vi "ScanSteuerung_to_Datapoints_Transposed.vi"(2 "Datapoints (-1=estimate)":i32=-1, 3 "ScanSteuerung":T3(array[cluster])=[{"Zeitpunkt [s]"=0.0, "Wirkung"=enum."Abs", "Kanal"=enum."GalvoX", "Wert (/s)"=-8.3466666667e-05}, {"Zeitpunkt [s]"=0.0, "Wirkung"=enum."Abs", "Kanal"=enum."GalvoY", "Wert (/s)"=6.7466666667e-05}, {"Zeitpunkt [s]"=0.0, "Wirkung"=enum."Inc", "Kanal"=enum."GalvoX", "Wert (/s)"=0.0888}, {"Zeitpunkt [s]"=0.0, "Wirkung"=enum."Inc", "Kanal"=enum."GalvoY", "Wert (/s)"=0.0}, {"Zeitpunkt [s]"=0.00119, "Wirkung"=enum."LoopStart", "Kanal"=enum."Loop", "Wert (/s)"=4.0}, {"Zeitpunkt [s]"=0.00119, "Wirkung"=enum."Abs", "Kanal"=enum."Digital", "Wert (/s)"=7.0}, {"Zeitpunkt [s]"=0.002, "Wirkung"=enum."Inc", "Kanal"=enum."GalvoX", "Wert (/s)"=-3.3095271315e-17}, {"Zeitpunkt [s]"=0.002, "Wirkung"=enum."Inc", "Kanal"=enum."GalvoY", "Wert (/s)"=-0.0818}, {"Zeitpunkt [s]"=0.0022, "Wirkung"=enum."Inc", "Kanal"=enum."GalvoX", "Wert (/s)"=-0.0888}, {"Zeitpunkt [s]"=0.0022, "Wirkung"=enum."Inc", "Kanal"=enum."GalvoY", "Wert (/s)"=0.0}, {"Zeitpunkt [s]"=0.00319, "Wirkung"=enum."Abs", "Kanal"=enum."Digital", "Wert (/s)"=5.0}, {"Zeitpunkt [s]"=0.0033900000000000002, "Wirkung"=enum."Abs", "Kanal"=enum."Digital", "Wert (/s)"=7.0}, {"Zeitpunkt [s]"=0.0042, "Wirkung"=enum."Inc", "Kanal"=enum."GalvoX", "Wert (/s)"=3.3095271315e-17}, {"Zeitpunkt [s]"=0.0042, "Wirkung"=enum."Inc", "Kanal"=enum."GalvoY", "Wert (/s)"=-0.0818}, {"Zeitpunkt [s]"=0.0044, "Wirkung"=enum."Inc", "Kanal"=enum."GalvoX", "Wert (/s)"=0.0888}, {"Zeitpunkt [s]"=0.0044, "Wirkung"=enum."Inc", "Kanal"=enum."GalvoY", "Wert (/s)"=0.0}, {"Zeitpunkt [s]"=0.00539, "Wirkung"=enum."Abs", "Kanal"=enum."Digital", "Wert (/s)"=5.0}, {"Zeitpunkt [s]"=0.00559, "Wirkung"=enum."LoopEnd", "Kanal"=enum."Loop", "Wert (/s)"=0.0}, {"Zeitpunkt [s]"=0.01879, "Wirkung"=enum."Abs", "Kanal"=enum."Digital", "Wert (/s)"=7.0}, {"Zeitpunkt [s]"=0.0196, "Wirkung"=enum."Inc", "Kanal"=enum."GalvoX", "Wert (/s)"=-3.3095271315e-17}, {"Zeitpunkt [s]"=0.0196, "Wirkung"=enum."Inc", "Kanal"=enum."GalvoY", "Wert (/s)"=-0.0818}, {"Zeitpunkt [s]"=0.0198, "Wirkung"=enum."Inc", "Kanal"=enum."GalvoX", "Wert (/s)"=-0.0888}, {"Zeitpunkt [s]"=0.0198, "Wirkung"=enum."Inc", "Kanal"=enum."GalvoY", "Wert (/s)"=0.0}, {"Zeitpunkt [s]"=0.02079, "Wirkung"=enum."Abs", "Kanal"=enum."Digital", "Wert (/s)"=5.0}, {"Zeitpunkt [s]"=0.02099, "Wirkung"=enum."Abs", "Kanal"=enum."Digital", "Wert (/s)"=7.0}, {"Zeitpunkt [s]"=0.0218, "Wirkung"=enum."Inc", "Kanal"=enum."GalvoX", "Wert (/s)"=0.0}, {"Zeitpunkt [s]"=0.0218, "Wirkung"=enum."Inc", "Kanal"=enum."GalvoY", "Wert (/s)"=0.0}, {"Zeitpunkt [s]"=0.0218, "Wirkung"=enum."LoopStart", "Kanal"=enum."Loop", "Wert (/s)"=2.0}, {"Zeitpunkt [s]"=0.021810000000000003, "Wirkung"=enum."Abs", "Kanal"=enum."GalvoX", "Wert (/s)"=-8.3466666667e-05}, {"Zeitpunkt [s]"=0.021810000000000003, "Wirkung"=enum."Abs", "Kanal"=enum."GalvoY", "Wert (/s)"=6.7466666667e-05}, {"Zeitpunkt [s]"=0.021810000000000003, "Wirkung"=enum."Inc", "Kanal"=enum."GalvoX", "Wert (/s)"=0.0888}, {"Zeitpunkt [s]"=0.021810000000000003, "Wirkung"=enum."Inc", "Kanal"=enum."GalvoY", "Wert (/s)"=0.0}, {"Zeitpunkt [s]"=0.023000000000000003, "Wirkung"=enum."LoopStart", "Kanal"=enum."Loop", "Wert (/s)"=4.0}, {"Zeitpunkt [s]"=0.023000000000000003, "Wirkung"=enum."Abs", "Kanal"=enum."Digital", "Wert (/s)"=7.0}, {"Zeitpunkt [s]"=0.023810000000000005, "Wirkung"=enum."Inc", "Kanal"=enum."GalvoX", "Wert (/s)"=-3.3095271315e-17}, {"Zeitpunkt [s]"=0.023810000000000005, "Wirkung"=enum."Inc", "Kanal"=enum."GalvoY", "Wert (/s)"=-0.0818}, {"Zeitpunkt [s]"=0.024010000000000004, "Wirkung"=enum."Inc", "Kanal"=enum."GalvoX", "Wert (/s)"=-0.0888}, {"Zeitpunkt [s]"=0.024010000000000004, "Wirkung"=enum."Inc", "Kanal"=enum."GalvoY", "Wert (/s)"=0.0}, {"Zeitpunkt [s]"=0.025, "Wirkung"=enum."Abs", "Kanal"=enum."Digital", "Wert (/s)"=5.0}, {"Zeitpunkt [s]"=0.025200000000000004, "Wirkung"=enum."Abs", "Kanal"=enum."Digital", "Wert (/s)"=7.0}, {"Zeitpunkt [s]"=0.026010000000000002, "Wirkung"=enum."Inc", "Kanal"=enum."GalvoX", "Wert (/s)"=3.3095271315e-17}, {"Zeitpunkt [s]"=0.026010000000000002, "Wirkung"=enum."Inc", "Kanal"=enum."GalvoY", "Wert (/s)"=-0.0818}, {"Zeitpunkt [s]"=0.026210000000000004, "Wirkung"=enum."Inc", "Kanal"=enum."GalvoX", "Wert (/s)"=0.0888}, {"Zeitpunkt [s]"=0.026210000000000004, "Wirkung"=enum."Inc", "Kanal"=enum."GalvoY", "Wert (/s)"=0.0}, {"Zeitpunkt [s]"=0.027200000000000002, "Wirkung"=enum."Abs", "Kanal"=enum."Digital", "Wert (/s)"=5.0}, {"Zeitpunkt [s]"=0.027400000000000004, "Wirkung"=enum."LoopEnd", "Kanal"=enum."Loop", "Wert (/s)"=0.0}, {"Zeitpunkt [s]"=0.040600000000000004, "Wirkung"=enum."Abs", "Kanal"=enum."Digital", "Wert (/s)"=7.0}, {"Zeitpunkt [s]"=0.04141, "Wirkung"=enum."Inc", "Kanal"=enum."GalvoX", "Wert (/s)"=-3.3095271315e-17}, {"Zeitpunkt [s]"=0.04141, "Wirkung"=enum."Inc", "Kanal"=enum."GalvoY", "Wert (/s)"=-0.0818}, {"Zeitpunkt [s]"=0.04161000000000001, "Wirkung"=enum."Inc", "Kanal"=enum."GalvoX", "Wert (/s)"=-0.0888}, {"Zeitpunkt [s]"=0.04161000000000001, "Wirkung"=enum."Inc", "Kanal"=enum."GalvoY", "Wert (/s)"=0.0}, {"Zeitpunkt [s]"=0.0426, "Wirkung"=enum."Abs", "Kanal"=enum."Digital", "Wert (/s)"=5.0}, {"Zeitpunkt [s]"=0.042800000000000005, "Wirkung"=enum."Abs", "Kanal"=enum."Digital", "Wert (/s)"=7.0}, {"Zeitpunkt [s]"=0.04361, "Wirkung"=enum."Inc", "Kanal"=enum."GalvoX", "Wert (/s)"=0.0}, {"Zeitpunkt [s]"=0.04361, "Wirkung"=enum."Inc", "Kanal"=enum."GalvoY", "Wert (/s)"=0.0}, {"Zeitpunkt [s]"=0.044789999999999996, "Wirkung"=enum."Abs", "Kanal"=enum."Digital", "Wert (/s)"=4.0}, {"Zeitpunkt [s]"=0.044800000000000006, "Wirkung"=enum."Abs", "Kanal"=enum."Digital", "Wert (/s)"=4.0}, {"Zeitpunkt [s]"=0.04361, "Wirkung"=enum."LoopEnd", "Kanal"=enum."Loop", "Wert (/s)"=0.0}, {"Zeitpunkt [s]"=0.06661, "Wirkung"=enum."Abs", "Kanal"=enum."Digital", "Wert (/s)"=0.0}], 4 "Aktiv":T2(array[ring])=[enum."GalvoX", enum."GalvoY"], 5 "Neues Zeitraster":dbl=1e-05) -> (0 "ScanSteuerungOut":T1(array[cluster])=[{"Zeitpunkt [s]"=0.0, "Wirkung"=enum."Abs", "Kanal"=0.0, "Wert (/s)"=0.0}, {"Zeitpunkt [s]"=0.0, "Wirkung"=enum."Inc", "Kanal"=0.0, "Wert (/s)"=0.0001}, {"Zeitpunkt [s]"=0.0, "Wirkung"=enum."Abs", "Kanal"=1.0, "Wert (/s)"=0.5}, {"Zeitpunkt [s]"=0.0, "Wirkung"=enum."IncInc", "Kanal"=0.0, "Wert (/s)"=-1.0000000000000002e-08}, {"Zeitpunkt [s]"=0.0, "Wirkung"=enum."IncInc", "Kanal"=1.0, "Wert (/s)"=-1.0000000000000002e-08}, {"Zeitpunkt [s]"=10000.0, "Wirkung"=enum."IncInc", "Kanal"=1.0, "Wert (/s)"=1.0000000000000002e-08}, {"Zeitpunkt [s]"=20000.0, "Wirkung"=enum."IncInc", "Kanal"=0.0, "Wert (/s)"=1.0000000000000002e-08}, {"Zeitpunkt [s]"=29999.999999999996, "Wirkung"=enum."IncInc", "Kanal"=1.0, "Wert (/s)"=-1.0000000000000002e-08}, {"Zeitpunkt [s]"=40000.0, "Wirkung"=enum."IncInc", "Kanal"=0.0, "Wert (/s)"=0.0}], 1 "Waveform Graph":dbl[][](graph))   [LabVIEW 2011]
panel:
  out "wrong command oder - STOP":bool
  out "Datapoints":i32=40001
  # "Transposed Datapoints!"
  # "After the loop there has to be at lest one datapoint in one activ channel\nOrder: add abs and rel-values, generate pint, add inc, add incinc to inc\ne.g. at t there is inc: t+1 there is the second pont (t,t+1) with one inc!"
  # "now with incinc support!\nnow with nested loops support!"
  # "Error handling for wrong loops!\nbut there is no error out"
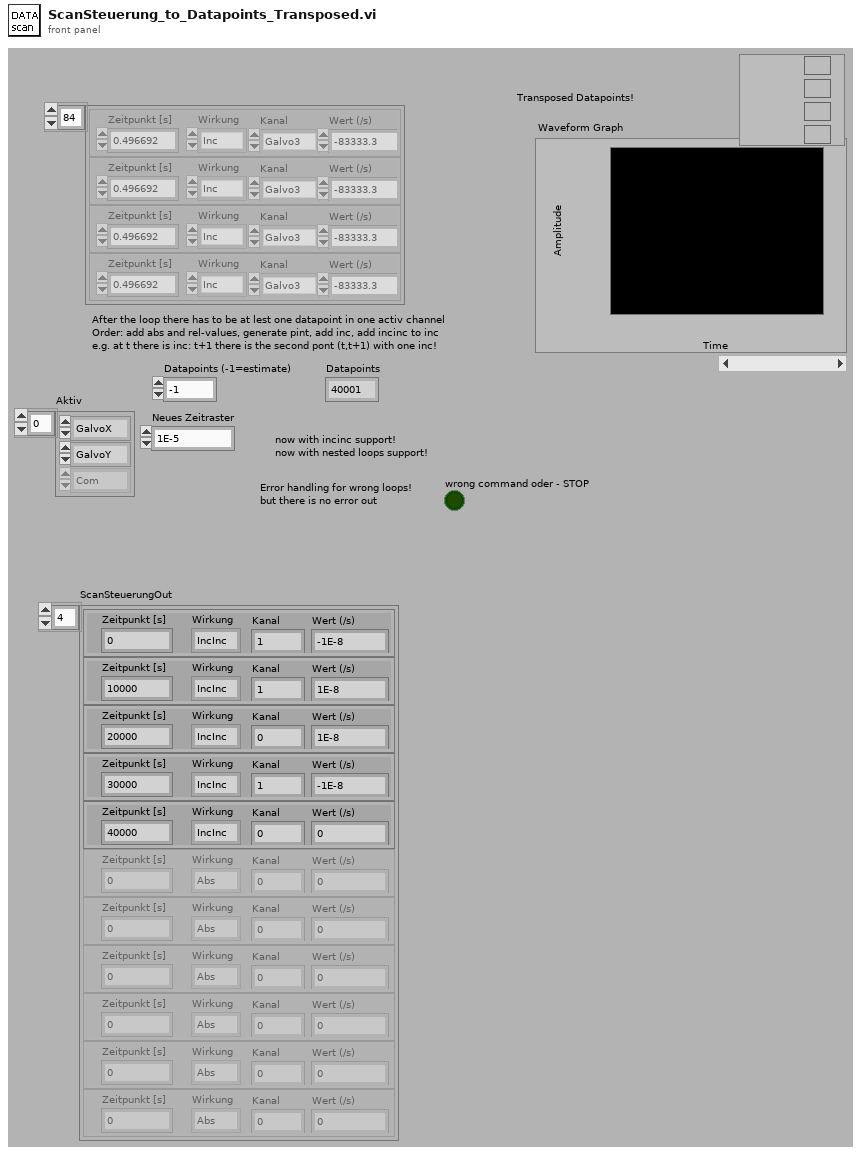
[diagram p1: front panel]
types:
  T1 = cluster{"Zeitpunkt [s]":dbl, "Wirkung":enum16{"Abs", "Rel", "Inc", "IncInc", "LoopStart", "LoopEnd"}, "Kanal":dbl, "Wert (/s)":dbl}[]
  T2 = enum16{"Com", "AnalogConfig", "AnalogValue", "GalvoX", "GalvoY", "Galvo3", "Galvo4", "Digital", "Free", "Loop", "SMoveTime", "Image1X", "Image1Y", "Image2X", "Image2Y"}[]
  T3 = cluster{"Zeitpunkt [s]":dbl, "Wirkung":enum16{"Abs", "Rel", "Inc", "IncInc", "LoopStart", "LoopEnd"}, "Kanal":enum16{"Com", "AnalogConfig", "AnalogValue", "GalvoX", "GalvoY", "Galvo3", "Galvo4", "Digital", "Free", "Loop", "SMoveTime", "Image1X", "Image1Y", "Image2X", "Image2Y"}, "Wert (/s)":dbl}[]
  T4 = cluster{"Time offsets":i32[], "Array":cluster{"Loopstart#":u32, "Loops to do":i32}[]}
  T5 = typedef "ScanControl.ctl" = cluster{"Time [s]":dbl, "action":T6, "channel":T7, "value (/s)":dbl}[]
  T6 = typedef "ScanControl_Action.ctl" = enum16{"Abs", "Rel", "Inc", "IncInc", "LoopStart", "LoopEnd", "WaitTriggerRising"}
  T7 = typedef "ScanControl_Channel.ctl" = enum16{"Com", "AnalogConfig", "AnalogValue", "GalvoX", "GalvoY", "Galvo3", "Galvo4", "Digital", "Free", "Loop", "SMoveTime", "Image1X", "Image1Y", "Image2X", "Image2Y"}
  T8 = cluster{"Zeitpunkt [s]":dbl, "Wirkung":enum16{"Abs", "Rel", "Inc", "IncInc", "LoopStart", "LoopEnd"}, "Kanal":i32, "Wert (/s)":dbl}[]
  T9 = cluster{"Zeitpunkt [s]":dbl, "Wirkung":enum16{"Abs", "Rel", "Inc", "IncInc", "LoopStart", "LoopEnd"}, "Kanal":i32, "Wert (/s)":dbl}
  T10 = enum16{"Abs", "Rel", "Inc", "IncInc", "LoopStart", "LoopEnd"}
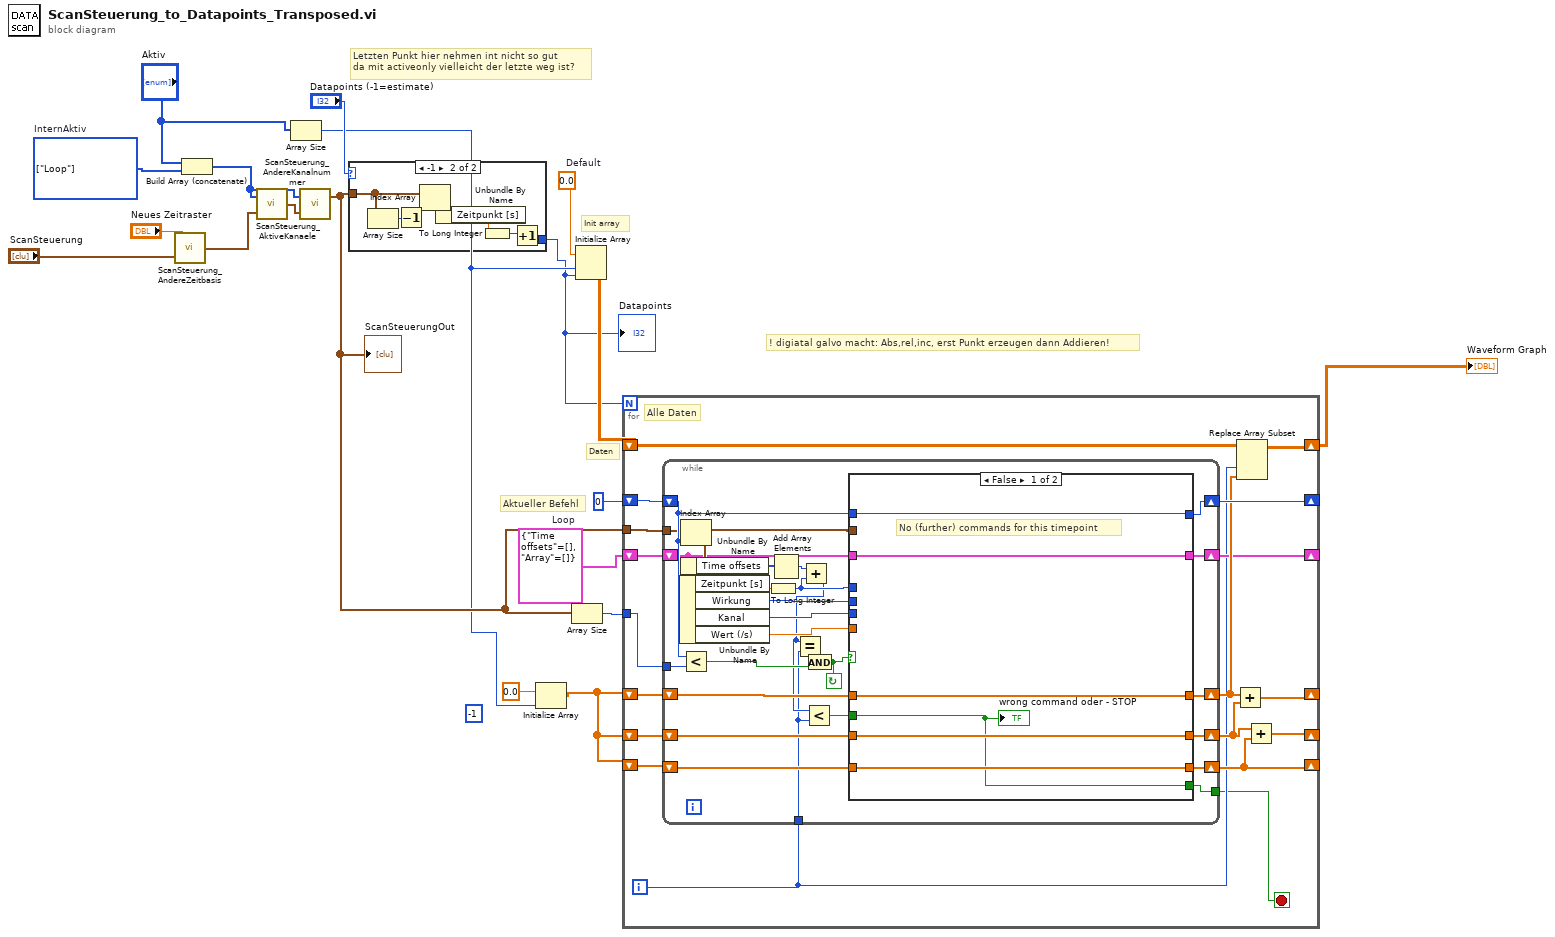
[diagram p0: block diagram]
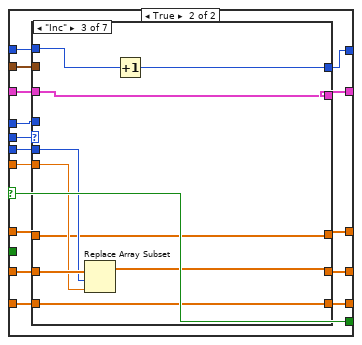
[diagram p3: hidden frame]
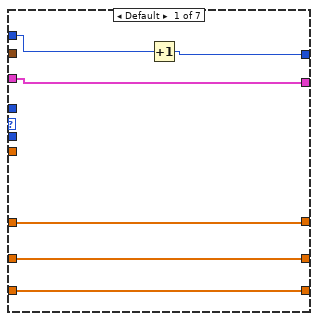
[diagram p4: hidden frame]
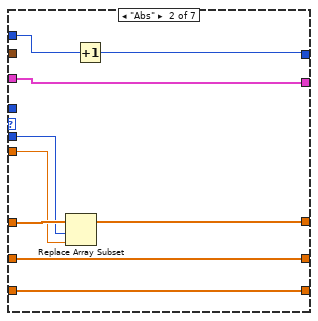
[diagram p5: hidden frame]
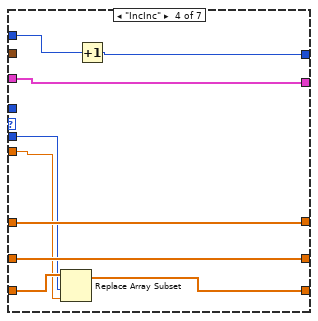
[diagram p6: hidden frame]
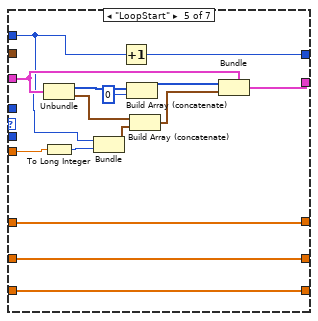
[diagram p7: hidden frame]
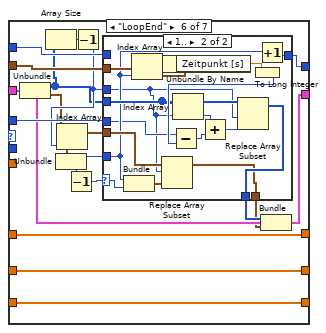
[diagram p8: hidden frame]
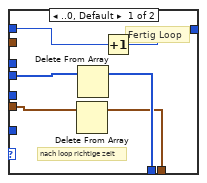
[diagram p9: hidden frame]
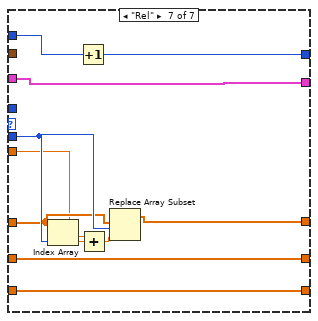
[diagram p10: hidden frame]
diagram:
  (unwired) -1 ("LoopLevel")
  w3 = T4 {"Time offsets"=[], "Array"=[]}  # Loop
  w12 = T2 [enum."Loop"] items=["Com", "AnalogConfig", "AnalogValue", "GalvoX", "GalvoY", "Galvo3", "Galvo4", "Digital", "Free", "Loop", "SMoveTime", "Image1X", "Image1Y", "Image2X", "Image2Y"]  # InternAktiv
  w19 = 0.0  # Default
  # "! digiatal galvo macht: Abs,rel,inc, erst Punkt erzeugen dann Addieren!"
  # "Letzten Punkt hier nehmen int nicht so gut\nda mit activeonly vielleicht der letzte weg ist?"
  # "Aktueller Befehl"
  # "Daten"
  # "Init array"
  n1 = call "ScanSteuerung_AndereZeitbasis.vi"("ScanSteuerung"="ScanSteuerung", "Neues Zeitraster"="Neues Zeitraster") -> ("ScanSteuerungOut"=w9:T5)
  n2 = Build Array (concatenate)("Aktiv", w12) -> (w10:T2)
  n3 = call "ScanSteuerung_AktiveKanaele.vi"("ScanSteuerung"=w9, "Aktiv"=w10) -> ("ScanSteuerungOut"=w14:T5)
  n4 = Array Size(array="Aktiv") -> (size(s)=w2:i32)
  n5 = call "ScanSteuerung_AndereKanalnummer.vi"("ScanSteuerung"=w14, "Neue Kanalnummer (nicht gefunden gibt 0!)"=w10) -> ("ScanSteuerungOut"=w13:T8)  [unwired: 1 out]
  "ScanSteuerungOut" <- w13
  n6 = case shown="-1" "Datapoints (-1=estimate)" {
    selector: "Datapoints (-1=estimate)" -> [w20 _]
    tunnel: w13 -> [_ w23]
    tunnel: [w20 w21] -> w1
    frame 0, Default {
    }
    frame -1 {
      n7 = Array Size(array=w23) -> (size(s)=w27:i32)
      n8 = Decrement(x=w27) -> (x-1=w26:i32)
      n9 = Index Array(array=w23, index=w26) -> (element=w25:T9)
      n10 = Unbundle By Name(w25) -> ("Zeitpunkt [s]"=w24:dbl)
      n11 = To Long Integer(number=w24) -> (32bit integer=w22:i32)
      n12 = Increment(x=w22) -> (x+1=w21:i32)
    }
  }
  "Datapoints" <- w1
  n13 = Initialize Array(0.0 ("element"), w2) -> (w4:dbl[])
  n14 = Array Size(array=w13) -> (size(s)=w16:i32)
  n15 = Initialize Array(w19, w2, w1) -> (w17:dbl[][])
  n16 = for {
    N: w1 -> [_]
    shift-left: w4 -> [w43]
    shift-right: [w39] -> _
    tunnel: w16 -> [w37]
    shift-left: u32 0 -> [w44]
    shift-right: [w38] -> _
    shift-left: w17 -> [w41]
    shift-right: [w40] -> w7
    tunnel: w13 -> [w45]
    shift-right: [w34] -> _
    shift-left: w4 -> [w42]
    shift-right: [w32] -> _
    shift-left: w4 -> [w35]
    shift-right: [w30] -> _
    shift-left: w3 -> [w31]
    i -> [w29]
    stop <- w28 stop-if-true
    # "Alle Daten"
    n17 = while {
      tunnel: w45 -> [w54]
      shift-right: [w64] -> w38
      shift-left: w44 -> [w61]
      shift-right: [w67] -> w36
      shift-left: w43 -> [w71]
      shift-right: [w66] -> w33
      shift-left: w42 -> [w70]
      tunnel: w29 -> [w48]
      tunnel: w37 -> [w60]
      shift-right: [w55] -> w32
      shift-left: w35 -> [w56]
      shift-right: [w52] -> w30
      shift-left: w31 -> [w53]
      tunnel: [w46] -> w28
      stop <- w57 continue-if-true
      n18 = Index Array(array=w54, index=w61) -> (element=w72:T9)
      n19 = Unbundle By Name(w72) -> ("Zeitpunkt [s]"=w63:dbl, "Wirkung"=w65:T10, "Kanal"=w69:i32, "Wert (/s)"=w68:dbl)
      n20 = Unbundle By Name(w53) -> ("Time offsets"=w51:i32[])
      n21 = Less?(x=w61, y=w60) -> (x < y?=w58:bool)
      n22 = To Long Integer(number=w63) -> (32bit integer=w62:i32)
      n23 = Add Array Elements(numeric array=w51) -> (sum=w50:i32)
      n24 = Add(x=w50, y=w62) -> (x+y=w49:i32)
      n25 = Equal?(x=w49, y=w48) -> (x = y?=w59:bool)
      n26 = Less?(x=w49, y=w48) -> (x < y?=w47:bool)
      n27 = And(x=w59, y=w58) -> (x .and. y?=w57:bool)
      n28 = case shown="False" w57 {
        selector: w57 -> [_ w79]
        tunnel: w71 -> [w78 w94]
        tunnel: w70 -> [w77 w93]
        tunnel: w69 -> [_ w92]
        tunnel: w68 -> [_ w91]
        tunnel: [w78 w90] -> w67
        tunnel: [w77 w89] -> w66
        tunnel: w65 -> [_ w88]
        tunnel: w61 -> [w76 w87]
        tunnel: [w76 w86] -> w64
        tunnel: w62 -> [_ w85]
        tunnel: w56 -> [w75 w84]
        tunnel: [w75 w83] -> w55
        tunnel: w54 -> [_ w82]
        tunnel: w53 -> [w74 w81]
        tunnel: [w74 w80] -> w52
        tunnel: w47 -> [w73 _]
        tunnel: [w73 w79] -> w46
        frame False {
          # "No (further) commands for this timepoint"
          "wrong command oder - STOP" <- w73
        }
        frame True {
          n29 = case shown="\"Inc\"" w88 {
            tunnel: w94 -> [w98 w109 w114 w127 w142 w161 w192]
            tunnel: w93 -> [w97 w105 w118 w126 w141 w160 w191]
            tunnel: w92 -> [_ w108 w116 w122 _ _ w193]
            tunnel: w91 -> [_ w107 w115 w121 w140 _ w190]
            tunnel: [w98 w106 w114 w127 w142 w161 w195] -> w90
            tunnel: [w97 w105 w117 w126 w141 w160 w191] -> w89
            tunnel: w87 -> [w100 w104 w113 w125 w135 w158 w188]
            tunnel: [w95 w103 w112 w124 w139 w159 w187] -> w86
            tunnel: w85 -> [_ _ _ _ _ w157 _]
            tunnel: w84 -> [w96 w102 w111 w123 w138 w156 w186]
            tunnel: [w96 w102 w111 w120 w138 w156 w186] -> w83
            tunnel: w82 -> [_ _ _ _ _ w155 _]
            tunnel: w81 -> [w99 w101 w110 w119 w136 w151 w185]
            tunnel: [w99 w101 w110 w119 w137 w152 w185] -> w80
            frame Default {
              n30 = Increment(x=w100) -> (x+1=w95:u32)
            }
            frame "Abs" {
              n31 = Replace Array Subset(array=w109, new element=w107, index=w108) -> (w106:dbl[])
              n32 = Increment(x=w104) -> (x+1=w103:u32)
            }
            frame "Inc" {
              n33 = Replace Array Subset(array=w118, new element=w115, index=w116) -> (w117:dbl[])
              n34 = Increment(x=w113) -> (x+1=w112:u32)
            }
            frame "IncInc" {
              n35 = Replace Array Subset(array=w123, new element=w121, index=w122) -> (w120:dbl[])
              n36 = Increment(x=w125) -> (x+1=w124:u32)
            }
            frame "LoopStart" {
              n37 = Unbundle(w136) -> ("Time offsets"=w129:i32[], "Array"=w128:cluster{"Loopstart#":u32, "Loops to do":i32}[])
              n38 = To Long Integer(number=w140) -> (32bit integer=w134:i32)
              n39 = Bundle(w135, w134) -> (w132:cluster{u32, i32})  [unwired: 1 out]
              n40 = Increment(x=w135) -> (x+1=w139:u32)
              n41 = Build Array (concatenate)(w129, 0) -> (w131:i32[])
              n42 = Build Array (concatenate)(w128, w132) -> (w133:cluster{"Loopstart#":u32, "Loops to do":i32}[])
              n43 = Bundle(cluster=w136, "Time offsets"=w131, "Array"=w133) -> (w137:T4)
            }
            frame "LoopEnd" {
              n44 = Unbundle(w151) -> ("Time offsets"=w144:i32[], "Array"=w143:cluster{"Loopstart#":u32, "Loops to do":i32}[])
              n45 = Array Size(array=w144) -> (size(s)=w146:i32)
              n46 = Decrement(x=w146) -> (x-1=w145:i32)
              n47 = Index Array(array=w143, index=w145) -> (element=w150:cluster{"Loopstart#":u32, "Loops to do":i32})
              n48 = Unbundle(w150) -> ("Loopstart#"=w153:u32, "Loops to do"=w154:i32)
              n49 = Decrement(x=w154) -> (x-1=w149:i32)
              n50 = case shown="1.." w149 {
                selector: w149 -> [_ w171]
                tunnel: w144 -> [w165 w175]
                tunnel: [w166 w184] -> w159
                tunnel: w158 -> [w167 _]
                tunnel: w157 -> [_ w169]
                tunnel: w155 -> [_ w182]
                tunnel: w153 -> [_ w170]
                tunnel: w145 -> [_ w168]
                tunnel: [w164 w176] -> w148
                tunnel: w143 -> [w163 w173]
                tunnel: [w162 w174] -> w147
                frame ..0, Default {
                  # "nach loop richtige zeit"
                  # "Fertig Loop"
                  n51 = Delete From Array(array=w163) -> (array with subset deleted=w162:cluster{"Loopstart#":u32, "Loops to do":i32}[])  [unwired: 2 in, 1 out]
                  n52 = Delete From Array(array=w165) -> (array with subset deleted=w164:i32[])  [unwired: 2 in, 1 out]
                  n53 = Increment(x=w167) -> (x+1=w166:u32)
                }
                frame 1.. {
                  n54 = Bundle("Loopstart#"=w170, w171) -> (w172:cluster{"Loopstart#":u32, i32})  [unwired: 1 out]
                  n55 = Index Array(array=w182, index=w170) -> (element=w181:T9)
                  n56 = Unbundle By Name(w181) -> ("Zeitpunkt [s]"=w180:dbl)
                  n57 = Replace Array Subset(array=w173, new element=w172, index=w168) -> (w174:cluster{"Loopstart#":u32, "Loops to do":i32}[])
                  n58 = Index Array(array=w175, index=w168) -> (element=w178:i32)
                  n59 = To Long Integer(number=w180) -> (32bit integer=w179:i32)
                  n60 = Subtract(x=w169, y=w179) -> (x-y=w183:i32)
                  n61 = Add(x=w178, y=w183) -> (x+y=w177:i32)
                  n62 = Replace Array Subset(array=w175, new element=w177, index=w168) -> (w176:i32[])
                  n63 = Increment(x=w170) -> (x+1=w184:u32)
                }
              }
              n64 = Bundle(cluster=w151, "Time offsets"=w148, "Array"=w147) -> (w152:T4)
            }
            frame "Rel" {
              n65 = Index Array(array=w192, index=w193) -> (element=w189:dbl)
              n66 = Increment(x=w188) -> (x+1=w187:u32)
              n67 = Add(x=w190, y=w189) -> (x+y=w194:dbl)
              n68 = Replace Array Subset(array=w192, new element=w194, index=w193) -> (w195:dbl[])
            }
          }
        }
      }
    }
    n69 = Add(x=w36, y=w33) -> (x+y=w39:dbl[])
    n70 = Replace Array Subset(array=w41, new element=w36, index (col)=w29) -> (w40:dbl[][])  [unwired: 1 in]
    n71 = Add(x=w33, y=w32) -> (x+y=w34:dbl[])
  }
  "Waveform Graph" <- w7
